vi "Set RIO INI Key.vi"(8 "error in":errorcluster, 11 "VS Engine Interface in":refnum<class "VS Engine Interface.lvclass">) -> (0 "error out":errorcluster, 2 "configuration file path":path, 3 "VS Engine Interface out":refnum<class "VS Engine Interface.lvclass">)   [LabVIEW 2024, in "VS Engine Abstraction.lvlib" / "VS Engine Interface.lvclass"]
uses:
  VS Engine Interface.lvclass
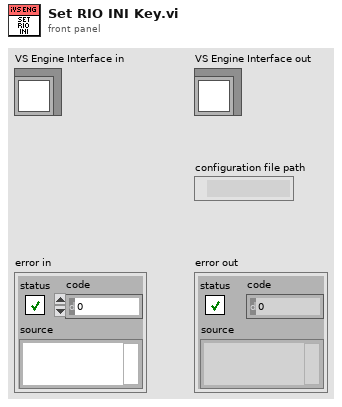
[diagram p1: front panel]
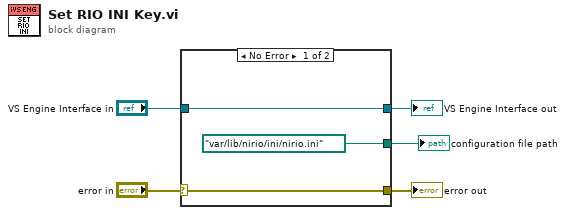
[diagram p0: block diagram]
diagram:
  n1 = case shown="No Error" "error in" {
    selector: "error in" -> [w8 w10]
    tunnel: [w8 w10] -> w4
    tunnel: [w7 w9] -> w2
    tunnel: "VS Engine Interface in" -> [w7 w9]
    tunnel: [path "/var/lib/nirio/ini/nirio.ini" ("configuration file path") _] -> w1
    frame No Error {
    }
    frame Error {
    }
  }
  "error out" <- w4
  "VS Engine Interface out" <- w2
  "configuration file path" <- w1
